vi "Function.vi"(8 "error in (no error)":errorcluster, 10 "Boolean A":bool, 11 "NOT in":refnum<class "NOT_Bool.lvclass">) -> (0 "error out":errorcluster, 2 "Boolean":bool, 3 "NOT out":refnum<class "NOT_Bool.lvclass">)   [LabVIEW 2021, in "NOT_Bool.lvclass"]
uses:
  NOT_Bool.lvclass
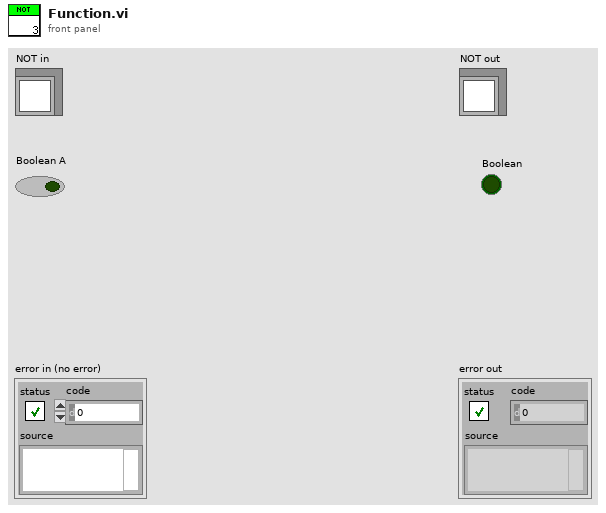
[diagram p1: front panel]
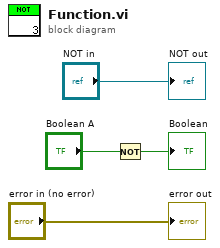
[diagram p0: block diagram]
diagram:
  n1 = Not(x="Boolean A") -> (.not. x?=→"Boolean":bool)
  "error out" <- "error in (no error)"
  "NOT out" <- "NOT in"
